vi "Continue Feedback.vi"(6 "error in (no error)":errorcluster, 7 "notification":dbl[](array[numeric]), 8 "Feedback Queue":refnum<queue>, 9 "Feedback State In":T1 {"Feedback Parameters"."Error Signal Source" items=["External Input", "APD Signal"]}) -> (0 "error out":errorcluster, 3 "Feedback State Out":T1 {"Feedback Parameters"."Error Signal Source" items=["External Input", "APD Signal"]})   [LabVIEW 2013, in "Feedback.lvlib"]
uses:
  Feedback.lvlib
  support/Message Queue/Message Cluster.ctl
  Feedback State.ctl
  Feedback Parameters.ctl
  Scan Parameters.ctl
  support/Message Queue/Enqueue Message (Single).vi
  support/Message Queue/Message Queue.lvlib
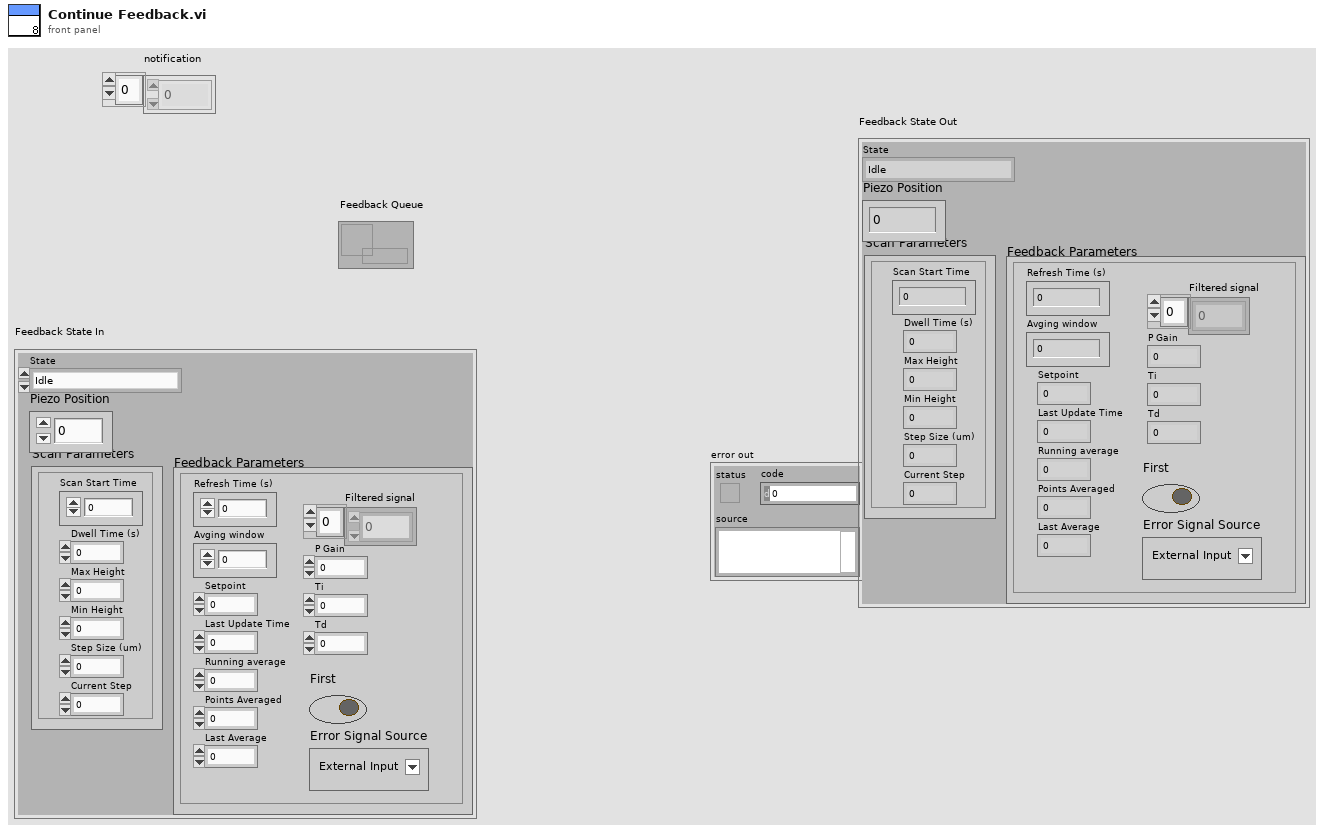
[diagram p1: front panel]
types:
  T1 = typedef "Feedback.lvlib/Feedback State.ctl" = cluster{"State":enum16{"Idle", "Feedback", "Scanning", "Averaging"}, "Feedback Parameters":T2, "Scan Parameters":T3, "Piezo Position":dbl}
  T2 = typedef "Feedback.lvlib/Feedback Parameters.ctl" = cluster{"Refresh Time (s)":dbl, "P Gain":dbl, "Setpoint":dbl, "Last Update Time":dbl, "Running average":dbl, "Points Averaged":dbl, "Last Average":dbl, "Filtered signal":dbl[], "Avging window":dbl, "Ti":dbl, "Td":dbl, "First":bool, "Error Signal Source":u16}
  T3 = typedef "Feedback.lvlib/Scan Parameters.ctl" = cluster{"Scan Start Time":dbl, "Step Size (um)":dbl, "Min Height":dbl, "Max Height":dbl, "Dwell Time (s)":dbl, "Current Step":dbl}
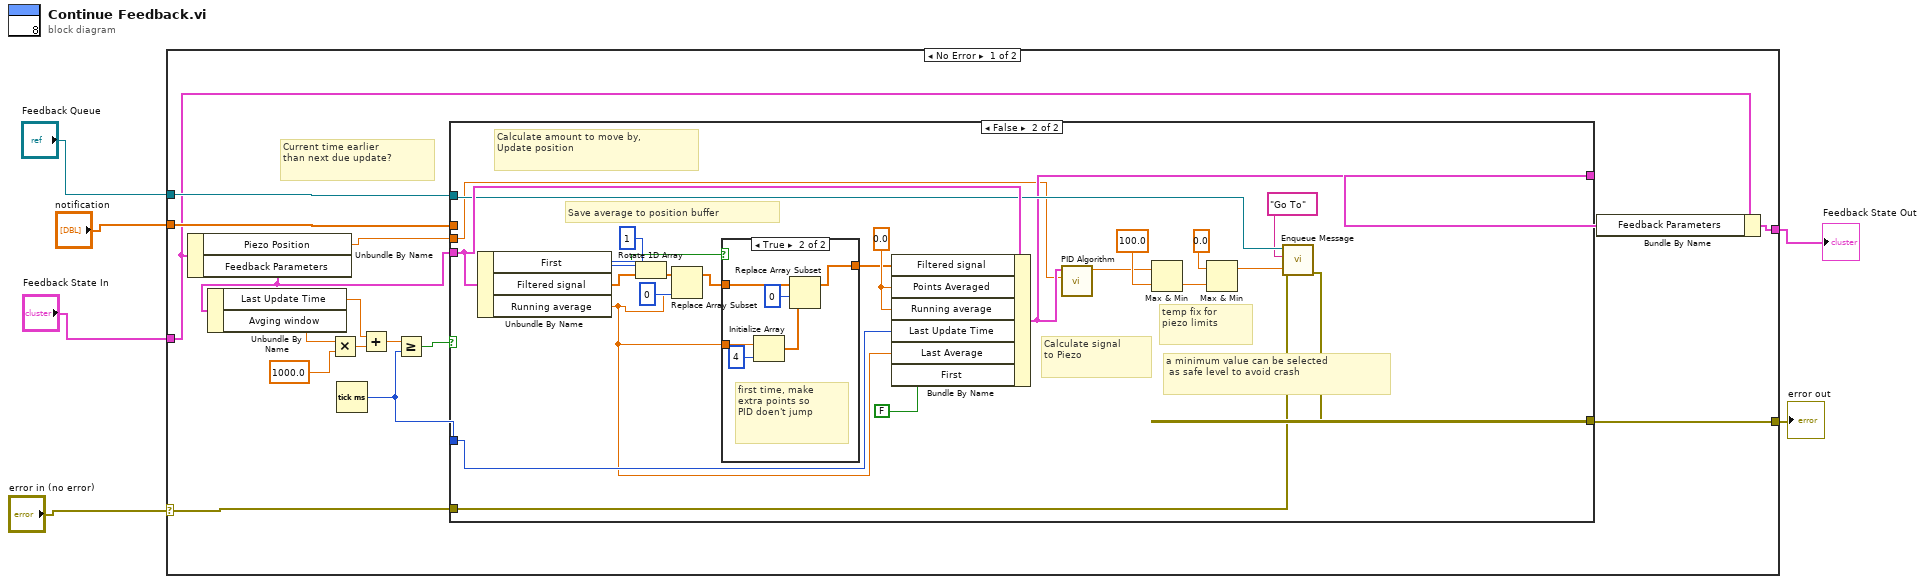
[diagram p0: block diagram]
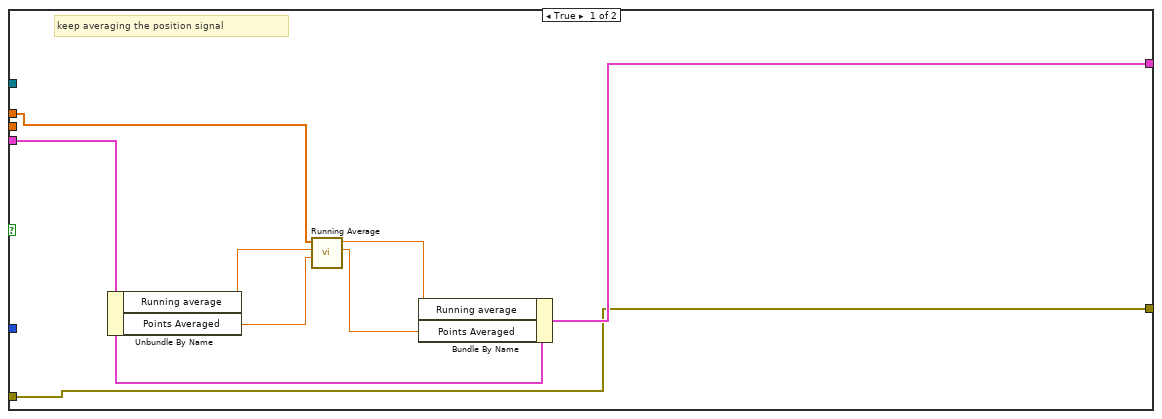
[diagram p2: hidden frame]
diagram:
  n1 = case shown="No Error" "error in (no error)" {
    selector: "error in (no error)" -> [w13 w62]
    tunnel: [w12 w62] -> w5
    tunnel: "Feedback State In" -> [w8 w61]
    tunnel: "notification" -> [w16 _]
    tunnel: [w10 w61] -> w3
    tunnel: "Feedback Queue" -> [w14 _]
    frame No Error {
      # "Current time earlier\nthan next due update?"
      n2 = Unbundle By Name(w8) -> ("Piezo Position"=w7:dbl, "Feedback Parameters"=w11:T2)
      n3 = Unbundle By Name(w11) -> ("Last Update Time"=w19:dbl, "Avging window"=w22:dbl)
      n4 = Multiply(x=w22, y=1000.0) -> (x*y=w20:dbl)
      n5 = Tick Count (ms)() -> (millisecond timer value=w15:u32)
      n6 = Add(x=w19, y=w20) -> (x+y=w18:dbl)
      n7 = Greater Or Equal?(x=w18, y=w15) -> (x >= y?=w17:bool)
      n8 = case shown="False" w17 {
        tunnel: w11 -> [w30 w51]
        tunnel: [w29 w38] -> w9
        tunnel: w16 -> [w27 _]
        tunnel: w15 -> [_ w52]
        tunnel: w14 -> [_ w50]
        tunnel: w13 -> [w28 w48]
        tunnel: [w28 w47] -> w12
        tunnel: w7 -> [_ w37]
        frame True {
          # "keep averaging the position signal"
          n9 = Unbundle By Name(w30) -> ("Running average"=w26:dbl, "Points Averaged"=w25:dbl)
          n10 = call "Running Average.vi"("Points Averaged"=w25, "Running average"=w26, "notification"=w27) -> ("Points Avged Out"=w24:dbl, "Running Avg Out"=w23:dbl)  [unwired: 7 in]
          n11 = Bundle By Name(cluster=w30, "Running average"=w23, "Points Averaged"=w24) -> (w29:T2)
        }
        frame False {
          w53 = 0.0 ("Feedback Parameters.Points Averaged")
          # "a minimum value can be selected\n as safe level to avoid crash"
          # "Calculate signal\nto Piezo"
          # "Save average to position buffer"
          # "temp fix for \npiezo limits"
          # "Calculate amount to move by,\nUpdate position"
          n12 = Unbundle By Name(w51) -> ("First"=w35:bool, "Filtered signal"=w42:dbl[], "Running average"=w31:dbl)
          n13 = Rotate 1D Array(1:w42, 2:1 ("n")) -> (0:w40:dbl[])
          n14 = Replace Array Subset(array=w40, new element=w31, index=0) -> (w33:dbl[])
          n15 = case shown="True" w35 {
            tunnel: w33 -> [w54 w60]
            tunnel: [w54 w59] -> w32
            tunnel: w31 -> [_ w58]
            frame False {
            }
            frame True {
              # "first time, make\nextra points so\nPID doen't jump"
              n16 = Initialize Array(w58, 4 ("dimension size")) -> (w55:dbl[])
              n17 = Replace Array Subset(array=w60, new element=w55, index=0) -> (w59:dbl[])
            }
          }
          n18 = Bundle By Name(cluster=w51, "Filtered signal"=w32, "Points Averaged"=w53, "Running average"=w53, "Last Update Time"=w52, "Last Average"=w31, "First"=FALSE) -> (w38:T2)
          n19 = call "PID Algorithm.vi"("Piezo Position"=w37, "Feedback Parameters"=w38) -> ("Signal to Piezo"=w36:dbl)  [unwired: 9 in]
          n20 = Max & Min(x=w36, y=100.0) -> (min(x,y)=w45:dbl)  [unwired: 1 out]
          n21 = Max & Min(x=0.0, y=w45) -> (max(x,y)=w43:dbl)  [unwired: 1 out]
          n22 = call-poly "Enqueue Message.vi"("error in (no error)"=w48, "Message Data"=w43, "Message"="Go To", "Message Queue"=w50) -> ("error out"=w47:errorcluster)  [unwired: 6 in, 1 out]
        }
      }
      n23 = Bundle By Name(cluster=w8, "Feedback Parameters"=w9) -> (w10:T1)
    }
    frame Error {
    }
  }
  "error out" <- w5
  "Feedback State Out" <- w3
